vi "concatenate.vi"(6 "Numeric Control 2":dbl, 7 "Numeric Control":dbl, 9 "Numeric Control 3":dbl, 10 "Numeric Control 4":dbl, 11 "Numeric Control 5":dbl) -> (3 "String":string)   [LabVIEW 2017]
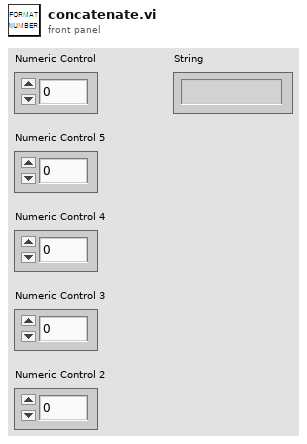
[diagram p1: front panel]
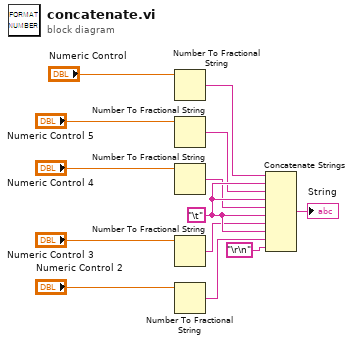
[diagram p0: block diagram]
diagram:
  w11 = "\t"
  n1 = Number To Fractional String(number="Numeric Control") -> (F-format string=w5:string)  [unwired: 3 in]
  n2 = Number To Fractional String(number="Numeric Control 5") -> (F-format string=w8:string)  [unwired: 3 in]
  n3 = Number To Fractional String(number="Numeric Control 4") -> (F-format string=w9:string)  [unwired: 3 in]
  n4 = Number To Fractional String(number="Numeric Control 3") -> (F-format string=w10:string)  [unwired: 3 in]
  n5 = Number To Fractional String(number="Numeric Control 2") -> (F-format string=w6:string)  [unwired: 3 in]
  n6 = Concatenate Strings(w5, w11, w8, w11, w9, w11, w10, w11, w6, "\r\n") -> (→"String":string)
